vi "PH_BL-Master.calc combined BL color.vi"(1 "Color State BL 2":i32, 2 "Color State BL 1":i32) -> (0 "Color State combined BL":i32)   [LabVIEW 2014, in "PH_BL-Master.lvlib"]
doc: "This calculates the color state after a combination of two beamlines; the combined output is\n\n1 if both input states are 1; else:\n6 if both input states are 6; else:\n3 if one or both input states are 3; else:\n0 if one ore both input states are 0; else:\n2"
uses:
  PH_BL-Master.lvlib
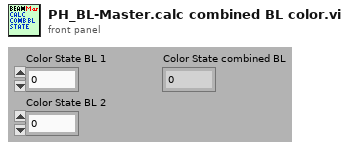
[diagram p1: front panel]
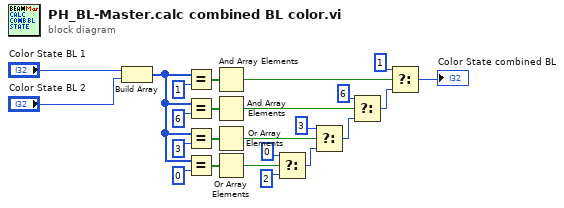
[diagram p0: block diagram]
diagram:
  n1 = Build Array("Color State BL 1", "Color State BL 2") -> (w19:i32[])
  n2 = Equal?(x=w19, y=1 ("Color State Exit fs-FE")) -> (x = y?=w4:bool[])
  n3 = Equal?(x=w19, y=6 ("Color State Exit fs-FE")) -> (x = y?=w9:bool[])
  n4 = Equal?(x=w19, y=3 ("Color State Exit fs-FE")) -> (x = y?=w14:bool[])
  n5 = Equal?(x=w19, y=0 ("Color State Exit fs-FE")) -> (x = y?=w20:bool[])
  n6 = And Array Elements(Boolean array=w4) -> (logical AND=w5:bool)
  n7 = And Array Elements(Boolean array=w9) -> (logical AND=w10:bool)
  n8 = Or Array Elements(Boolean array=w14) -> (logical OR=w15:bool)
  n9 = Or Array Elements(Boolean array=w20) -> (logical OR=w21:bool)
  n10 = Select(t=0 ("Color State Exit fs-FE"), s=w21, f=2) -> (s? t:f=w22:i32)
  n11 = Select(t=3 ("Color State Exit fs-FE"), s=w15, f=w22) -> (s? t:f=w16:i32)
  n12 = Select(t=6 ("Color State Exit fs-FE"), s=w10, f=w16) -> (s? t:f=w11:i32)
  n13 = Select(t=1 ("Color State Exit fs-FE"), s=w5, f=w11) -> (s? t:f=→"Color State combined BL":i32)
